vi "InitializeChop.vi"(8 "error in (no error)":errorcluster, 11 "VISA resource name":refnum<visa-resource-name>) -> (0 "error out":errorcluster, 3 "VISA resource name out":refnum<visa-resource-name>)   [LabVIEW 2017, in "LIAinteraction.lvlib"]
uses:
  LIAinteraction.lvlib
panel:
  out "Success?":bool=TRUE
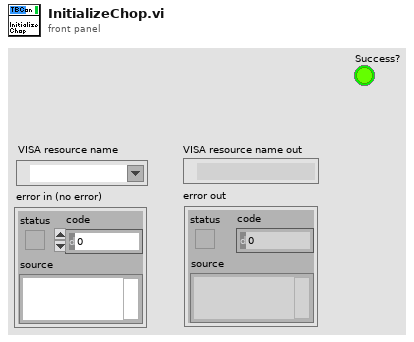
[diagram p1: front panel]
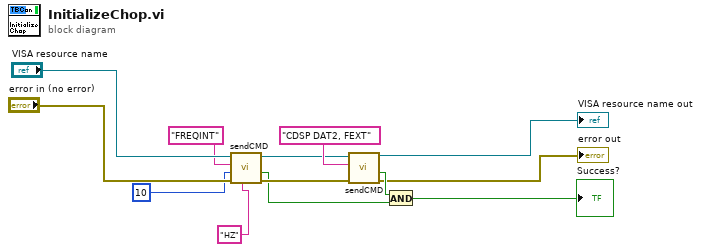
[diagram p0: block diagram]
diagram:
  n1 = call "sendCMD.vi"("Unit"="HZ", "error in (no error)"="error in (no error)", "Value"=10, "Command"="FREQINT", "VISA resource name"="VISA resource name") -> ("error out"=w8:errorcluster, "Success?"=w6:bool, "VISA resource name out"=w9:refnum<visa-resource-name>)  [unwired: 4 in]
  n2 = call "sendCMD.vi"("error in (no error)"=w8, "Command"="CDSP DAT2, FEXT", "VISA resource name"=w9) -> ("error out"=→"error out":errorcluster, "Success?"=w7:bool, "VISA resource name out"=→"VISA resource name out":refnum<visa-resource-name>)  [unwired: 6 in]
  n3 = And(x=w7, y=w6) -> (x .and. y?=→"Success?":bool)
